vi "Gamma_range.vi"(1 "Illuminant Table":string[][](array[string]), 2 "NumberOfRows":dbl) -> (0 "GammaInterval":dbl[](array[numeric]))   [LabVIEW 2014]
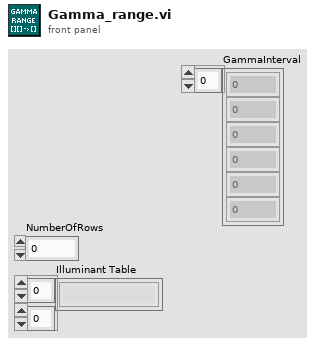
[diagram p1: front panel]
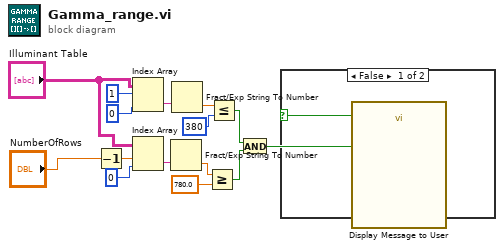
[diagram p0: block diagram]
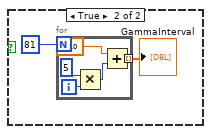
[diagram p2: hidden frame]
diagram:
  n1 = Decrement(x="NumberOfRows") -> (x-1=w14:dbl)
  n2 = Index Array(array="Illuminant Table", index (row)=1, index (col)=0) -> (element=w11:string)
  n3 = Index Array(array="Illuminant Table", index (row)=w14, index (col)=0 ("disabled index (col)")) -> (element=w10:string)
  n4 = Fract/Exp String To Number(string=w10) -> (number=w7:dbl)  [unwired: 3 in, 1 out]
  n5 = Fract/Exp String To Number(string=w11) -> (number=w4:dbl)  [unwired: 3 in, 1 out]
  n6 = Greater Or Equal?(x=w7, y=780.0) -> (x >= y?=w1:bool)
  n7 = Less Or Equal?(x=w4, y=380 ("x")) -> (x <= y?=w2:bool)
  n8 = And(x=w2, y=w1) -> (x .and. y?=w5:bool)
  n9 = case shown="False" w5 {
    frame False {
      n10 = call "Display Message to User"() -> ()  [unwired: 10 in, 2 out]
    }
    frame True {
      n11 = for {
        N: 81 -> [_]
        tunnel: [w19] -> w17 mode=indexing
        i -> [w21]
        n12 = Multiply(x=5, y=w21) -> (x*y=w22:i32)
        n13 = Add(x=380.0, y=w22) -> (x+y=w19:dbl)
      }
      "GammaInterval" <- w17
    }
  }
